vi "FisherPaykel Discover Motor Controllers.vi"(8 "error in (no error)":errorcluster) -> (0 "Error Out":errorcluster, 3 "Array":refnum<visa-resource-name>[](array[refnum]))   [LabVIEW 2016]
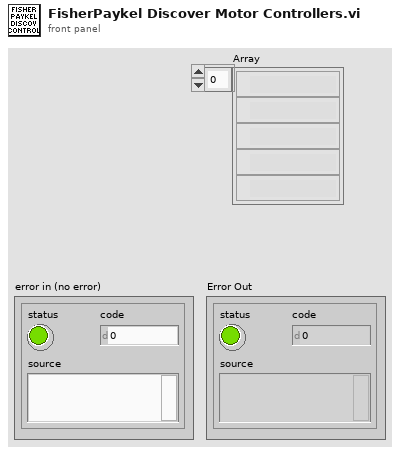
[diagram p1: front panel]
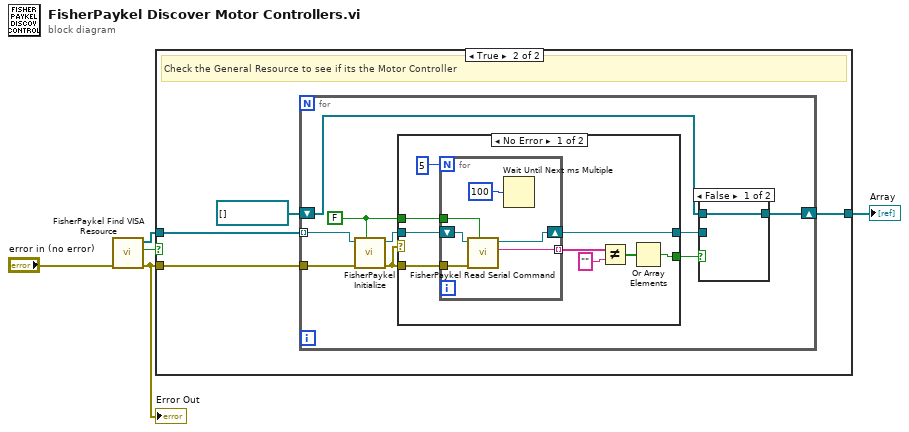
[diagram p0: block diagram]
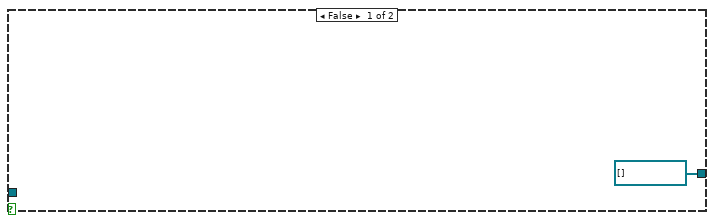
[diagram p2: hidden frame]
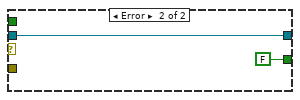
[diagram p3: hidden frame]
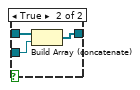
[diagram p4: hidden frame]
diagram:
  n1 = call "FisherPaykel Find VISA Resource.vi"("Error In"="error in (no error)") -> ("Error Out"=w1:errorcluster, "General Resource Found"=w2:bool, "VISA Resource"=w3:refnum<visa-resource-name>[])  [unwired: 8 in]
  "Error Out" <- w1
  n2 = case shown="True" w2 {
    tunnel: w3 -> [_ w10]
    tunnel: [refnum<visa-resource-name>[] [] w7] -> w5
    tunnel: w1 -> [_ w9]
    frame False {
    }
    frame True {
      # "Check the General Resource to see if its the Motor Controller"
      n3 = for {
        tunnel: w10 -> [w19] mode=indexing
        tunnel: w9 -> [w14]
        shift-right: [w11] -> w7
        shift-left: refnum<visa-resource-name>[] [] -> [w12]
        w17 = FALSE ("Debug")
        n4 = call "FisherPaykel Initialize.vi"("Debug"=w17, "Error In"=w14, "VISA Refnum in"=w19) -> ("Error Out"=w13:errorcluster, "VISA Refnum out"=w18:refnum<visa-resource-name>)  [unwired: 7 in]
        n5 = case shown="No Error" w13 {
          tunnel: w18 -> [w28 w36]
          tunnel: w13 -> [w20 _]
          tunnel: w17 -> [w27 _]
          tunnel: [w22 FALSE] -> w16
          tunnel: [w21 w36] -> w15
          frame No Error {
            n6 = for {
              N: 5 -> [_]
              tunnel: w27 -> [w33]
              tunnel: [w31] -> w24 mode=indexing
              shift-right: [w30] -> w21
              shift-left: w28 -> [w34]
              tunnel: w20 -> [w29]
              n7 = call "FisherPaykel Read Serial Command.vi"("Debug"=w33, "Error In"=w29, "VISA Refnum in"=w34) -> ("Serial Read Command"=w31:string, "VISA Refnum out"=w30:refnum<visa-resource-name>)  [unwired: 6 in, 1 out]
              n8 = Wait Until Next ms Multiple(millisecond multiple=u32 100) -> ()  [unwired: 1 out]
            }
            n9 = Not Equal?(x=w24, y="") -> (x != y?=w23:bool[])
            n10 = Or Array Elements(Boolean array=w23) -> (logical OR=w22:bool)
          }
          frame Error {
          }
        }
        n11 = case shown="False" w16 {
          tunnel: w15 -> [_ w39]
          tunnel: [w37 w38] -> w11
          tunnel: w12 -> [w37 w40]
          frame False {
          }
          frame True {
            n12 = Build Array (concatenate)(w40, w39) -> (w38:refnum<visa-resource-name>[])
          }
        }
      }
    }
  }
  "Array" <- w5
